vi "WebPublishing-DropIn.vi"(4 "Error In":errorcluster, 5 "Stop Occurrence":refnum<k4>, 6 "Mode (Snapshot)":enum16{"Snapshot", "Monitored", "Embedded"}(ring), 7 "VI Ref":refnum<vi>) -> (0 "Error Out":errorcluster, 1 "Web Server:Active":bool, 2 "URL":string, 3 "HTML File Name":path)   [LabVIEW 2016, in "CS++Utilities.lvlib"]
doc: "This VI will generate a Web Publishing HTML file for the Caller-VI in Web-Server file space to be viewed by remote Web-Browser.\n\nThis VI is used as drop-in. Simply connect an occurrence to stop this VI. It will clean up generated files.\n\n<b>Attention:</b> Library- and VI-Names should avoid any special charackters. They may be not recognizes by the Web-Publishing-Server."
uses:
  CS++Utilities.lvlib
panel:
  in  "Html_Code_Snapshot":string="<!DOCTYPE HTML PUBLIC \"-//W3C//DTD HTML 3.2 Draft//EN\">\n<HTML>\n<HEAD>\n<TITLE>WINDOW_TITLE</TITLE>\n</HEAD>\n<BODY >\n<H1>WINDOW_TITLE</H1>\n<IMG src=\"/.snap?SUBSTITUTE_VI_NAME\" alt=\"SUBSTITUTE_VI_NAME\" BORDER=1>\n<p>VI_DESCRIPTION</p>\n<p>HTML generated by CS++ WebPublishing-DropIn, H.Brand@gsi.de.</p>\n</BODY>\n</HTML>\n"
  in  "Html_Code_Monitor":string="<!DOCTYPE HTML PUBLIC \"-//W3C//DTD HTML 3.2 Draft//EN\">\n<HTML>\n<HEAD>\n<TITLE>WINDOW_TITLE</TITLE>\n<script language=\"javascript\">\n   <!-- \n   LVImages = new Array();\n   LVSrcs = new Array();\n   function LVSched(image, delay) {\n      LVImages[LVImages.length] = image;\n      LVSrcs[LVSrcs.length] = image.src;\n      setInterval(\"LVUpdate(\"+(LVImages.length-1)+\")\", delay);\n      image.onload='';\n   }\n   function LVUpdate(index) {\n      LVImages[index].src = LVSrcs[index] + '&' + Math.random();\n   }\n   //-->\n</script>\n</HEAD>\n<BODY >\n<H1>WINDOW_TITLE</H1>\n<IMG src=\"/.snap?SUBSTITUTE_VI_NAME\" alt=\"SUBSTITUTE_VI_NAME\" BORDER=1 onload=\"LVSched(this, 1000)\">\n<p>VI_DESCRIPTION</p>\n<p>HTML generated by CS++ WebPublishing-DropIn, H.Brand@gsi.de.</p>\n</BODY>\n</HTML>"
  in  "Html_Code_Embedded":string="<!DOCTYPE HTML PUBLIC \"-//W3C//DTD HTML 3.2 Draft//EN\">\n<HTML>\n<HEAD>\n<Script Language=\"JavaScript\">\nvar userAgent = navigator.userAgent;\nvar versionOffset = userAgent.indexOf(\"Chrome\");\n\nif (versionOffset != -1)\n{\n    var fullVersion = userAgent.substring(versionOffset+7);\n    var majorVersion = parseInt(''+fullVersion,10);\n    if (majorVersion >= 42)\n    {\n\tvar plugins = navigator.plugins;\n\tvar hasNIPlugin = false;\n\tfor (var i = 0; i < plugins.length; i++) {\n\t\tif (plugins[i].name.indexOf(\"National Instruments\") != -1) {\n\t\t\thasNIPlugin = true;\n\t\t}\n\t}\n\tif (hasNIPlugin == false) {\n        \tdocument.write('<strong><em>NI has detected that your ' +\n                               'browser might be blocking a plug-in.  '+\n                               'Visit ni.com/info and enter the following '+\n                               'Info Code for more information: '+\n                               'BlockedPlugin</em></strong>')\n\t}\n    }\n}\n</Script>\n<TITLE>WINDOW_TITLE</TITLE>\n</HEAD>\n<BODY >\n<H1>WINDOW_TITEL</H1>\n<p><TABLE BORDER=1 BORDERCOLOR = #000000><TR><TD>\n<OBJECT ID=\"LabVIEWControl\" CLASSID=\"CLSID:A40B0AD4-B50E-4E58-8A1D-8544233807B8\" WIDTH=PANEL_WIDTH HEIGHT=PANEL_HEIGHT CODEBASE=\"ftp://ftp.ni.com/support/labview/runtime/windows/2016/LVRTE2016min.exe\">\n<PARAM name=\"LVFPPVINAME\" value=\"SUBSTITUTE_VI_NAME\">\n<PARAM name=\"REQCTRL\" value=false>\n<EMBED SRC=\".LV_FrontPanelProtocol.rpvi160\" LVFPPVINAME=\"SUBSTITUTE_VI_NAME\" REQCTRL=false TYPE=\"application/x-labviewrpvi160\" WIDTH=PANEL_HEIGHT HEIGHT=PANEL_HEIGHT  PLUGINSPAGE=\"http://digital.ni.com/express.nsf/bycode/exck2m\">\n</EMBED>\n</OBJECT>\n</TD></TR></TABLE></p>\n<p>VI_DESCRIPTION</p>\n<p>HTML generated by CS++ WebPublishing-DropIn, H.Brand@gsi.de.</p>\n</BODY>\n</HTML>"
  in  "SHDocVw.IWebBrowser2":refnum<k7>
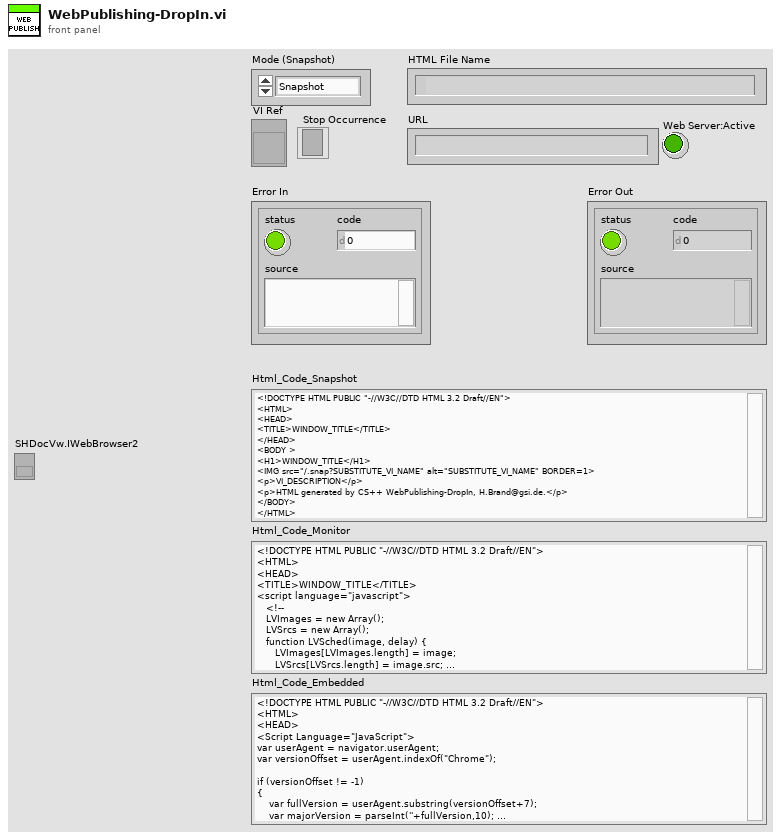
[diagram p1: front panel]
types:
  T1 = enum16{"open", "replace", "create", "open or create", "replace or create", "replace or create with confirmation"}
  T2 = typedef "LVRectTypeDef.ctl" = cluster{"Left":i16, "Top":i16, "Right":i16, "Bottom":i16}
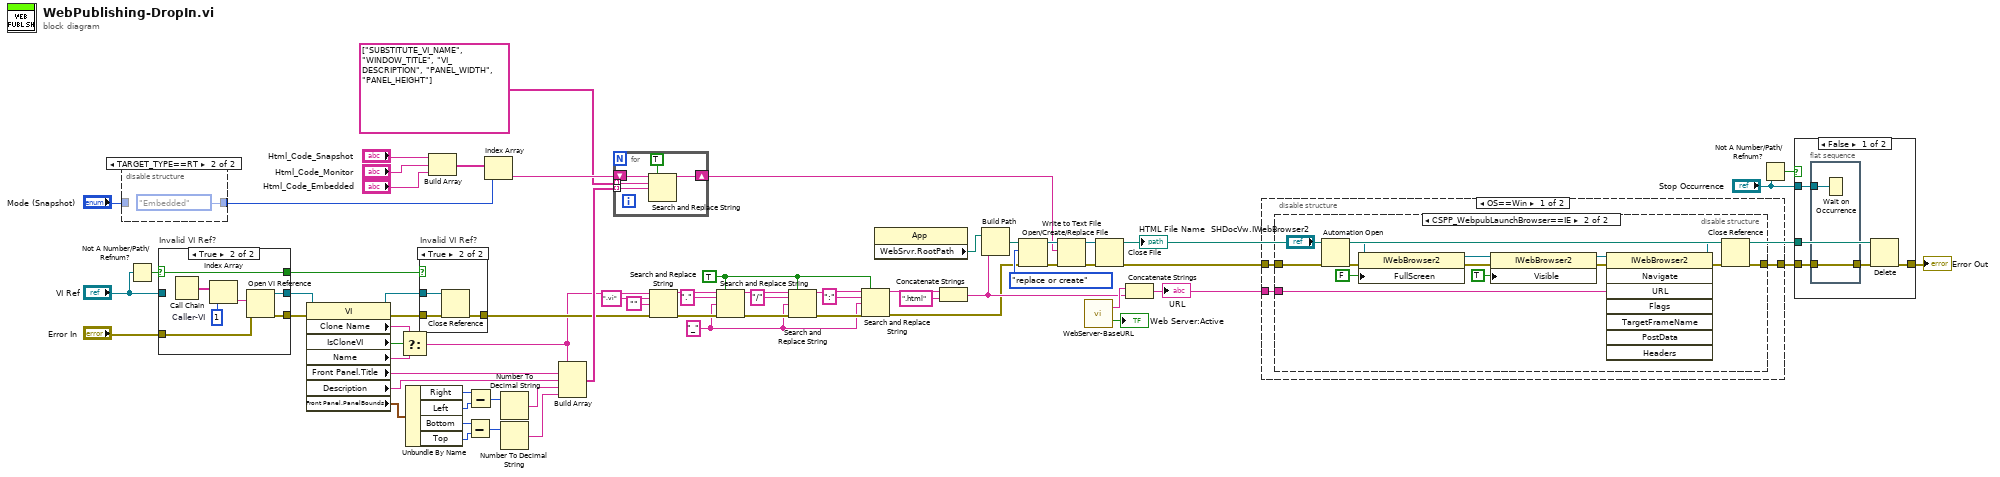
[diagram p0: block diagram]
diagram:
  w10 = TRUE ("replace all? (F)")
  w2 = "_"
  n1 = disable-structure shown="TARGET_TYPE==RT" {
    disable-tunnel: "Mode (Snapshot)" -> [w68 _]
    disable-tunnel: [w68 enum16{"Snapshot", "Monitored", "Embedded"}."Embedded" ("Mode (Snapshot)")] -> w26
    frame condition #0 (active) {
    }
    frame condition #1 {
    }
  }
  n2 = Not A Number/Path/Refnum?(number/path/refnum="VI Ref") -> (NaN/Path/Refnum?=w30:bool)
  n3 = case "Invalid VI Ref?" shown="True" w30 {
    selector: w30 -> [w70 w73]
    tunnel: [w72 w76] -> w67
    tunnel: [w71 w75] -> w61
    tunnel: "Error In" -> [w71 w74]
    tunnel: "VI Ref" -> [w72 _]
    tunnel: [w70 w73] -> w28
    frame False {
    }
    frame True {
      w79 = 1  # Caller-VI
      n4 = Call Chain() -> (call chain=w78:string[])
      n5 = Index Array(array=w78, index=w79) -> (element=w77:string)
      n6 = Open VI Reference(vi path=w77, error in (no error)=w74) -> (vi reference=w76:refnum<vi>, error out=w75:errorcluster)  [unwired: 4 in]
    }
  }
  n7 = property class="VI"(reference=w67, error in=w61) -> (reference out=w66:refnum<vi>, error out=w60:errorcluster, "Clone Name"=w45:string, "IsCloneVI"=w46:bool, "Name"=w44:string, "Front Panel.Title"=w23:string, "Description"=w22:string, "Front Panel.PanelBounds"=w20:T2)
  n8 = Select(t=w45, s=w46, f=w44) -> (s? t:f=w1:string)
  n9 = Unbundle By Name(w20) -> ("Right"=w19:i16, "Left"=w18:i16, "Bottom"=w17:i16, "Top"=w16:i16)
  n10 = case "Invalid VI Ref?" shown="True" w28 {
    tunnel: w66 -> [_ w83]
    tunnel: w60 -> [w80 w82]
    tunnel: [w80 w81] -> w5
    frame False {
    }
    frame True {
      n11 = Close Reference(reference=w83, error in (no error)=w82) -> (error out=w81:errorcluster)
    }
  }
  n12 = Build Array("Html_Code_Snapshot", "Html_Code_Monitor", "Html_Code_Embedded") -> (w52:string[])
  n13 = Subtract(x=w17, y=w16) -> (x-y=w13:i16)
  n14 = Subtract(x=w19, y=w18) -> (x-y=w15:i16)
  n15 = Index Array(array=w52, index=w26) -> (element=w51:string)
  n16 = Number To Decimal String(number=w13) -> (decimal integer string=w12:string)  [unwired: 1 in]
  n17 = Number To Decimal String(number=w15) -> (decimal integer string=w14:string)  [unwired: 1 in]
  n18 = Build Array(w1, w23, w22, w14, w12) -> (w24:string[])
  n19 = for {
    tunnel: string[] ["SUBSTITUTE_VI_NAME", "WINDOW_TITLE", "VI_DESCRIPTION", "PANEL_WIDTH", "PANEL_HEIGHT"] -> [w86] mode=indexing
    tunnel: w24 -> [w85] mode=indexing
    shift-right: [w84] -> w21
    shift-left: w51 -> [w87]
    n20 = Search and Replace String(replace all?=TRUE ("replace all? (F)"), input string=w87, search string=w86, replace string=w85) -> (result string=w84:string)  [unwired: 4 in, 3 out]
  }
  n21 = Search and Replace String(input string=w1, search string=".vi", replace string="", error in=w5) -> (result string=w3:string, error out=w4:errorcluster)  [unwired: 4 in, 2 out]
  n22 = Search and Replace String(replace all?=w10, input string=w3, search string=".", replace string=w2, error in=w4) -> (result string=w9:string, error out=w8:errorcluster)  [unwired: 3 in, 2 out]
  n23 = Search and Replace String(replace all?=w10, input string=w9, search string="/", replace string=w2, error in=w8) -> (result string=w32:string, error out=w31:errorcluster)  [unwired: 3 in, 2 out]
  n24 = Search and Replace String(replace all?=w10, input string=w32, search string=":", replace string=w2, error in=w31) -> (result string=w6:string, error out=w7:errorcluster)  [unwired: 3 in, 2 out]
  n25 = property class="App"() -> ("WebSrvr.RootPath"=w47:path)  [unwired: 2 in, 2 out]
  n26 = Concatenate Strings(w6, ".html") -> (w42:string)
  n27 = Build Path(base path=w47, name or relative path=w42) -> (appended path=w48:path)
  n28 = Open/Create/Replace File(file path (use dialog)=w48, error in=w7, operation (0:open)=T1."replace or create") -> (refnum out=w65:refnum<file>, error out=w63:errorcluster)  [unwired: 3 in, 1 out]
  n29 = Write to Text File(file (use dialog)=w65, text=w21, error in=w63) -> (refnum out=w64:refnum<file>, error out=w62:errorcluster)  [unwired: 1 in, 1 out]
  n30 = call "WebServer-BaseURL.vi"() -> ("Web Server:Active"=→"Web Server:Active":bool, "Web-Server:Base-URL"=w43:string)
  n31 = Close File(refnum=w64, error in=w62) -> (path=w38:path, error out=w56:errorcluster)
  "HTML File Name" <- w38
  n32 = Concatenate Strings(w43, w42) -> (w41:string)
  "URL" <- w41
  n33 = disable-structure shown="OS==Win" {
    disable-tunnel: w56 -> [w91 w106]
    disable-tunnel: w41 -> [w90 _]
    disable-tunnel: [w89 w106] -> w39
    frame condition #0 (active) {
      n34 = disable-structure shown="CSPP_WebpubLaunchBrowser==IE" {
        disable-tunnel: w91 -> [_ w105]
        disable-tunnel: w90 -> [_ w104]
        disable-tunnel: [_ w103] -> w89
        frame condition #0 {
        }
        frame condition #1 (active) {
          n35 = Automation Open(error in (no error)=w105, Automation Refnum="SHDocVw.IWebBrowser2") -> (Automation Refnum=w96:refnum<k7>, error out=w97:errorcluster)  [unwired: 2 in]
          n36 = property class="IWebBrowser2"(reference=w96, error in=w97, "FullScreen"=FALSE) -> (reference out=w101:refnum<k7>, error out=w102:errorcluster)
          n37 = property class="IWebBrowser2"(reference=w101, error in=w102, "Visible"=TRUE) -> (reference out=w94:refnum<k7>, error out=w95:errorcluster)
          n38 = invoke class="IWebBrowser2" method="Navigate"(reference=w94, error in=w95, "URL"=w104) -> (reference out=w92:refnum<k7>, error out=w93:errorcluster)  [unwired: 5 in, 6 out]
          n39 = Close Reference(reference=w92, error in (no error)=w93) -> (error out=w103:errorcluster)
        }
      }
    }
    frame condition #1 {
    }
  }
  n40 = Not A Number/Path/Refnum?(number/path/refnum="Stop Occurrence") -> (NaN/Path/Refnum?=w35:bool)
  n41 = case shown="False" w35 {
    tunnel: w39 -> [w110 w114]
    tunnel: w38 -> [w109 _]
    tunnel: [w108 w114] -> w37
    tunnel: "Stop Occurrence" -> [w107 _]
    frame False {
      n42 = flat-sequence {
        tunnel: [w113] -> w111
        tunnel: w110 -> [w113]
        tunnel: w107 -> [w112]
        frame #0 {
          n43 = Wait on Occurrence(2:w112) -> ()  [unwired: 2 in, 1 out]
        }
      }
      n44 = Delete(path (use dialog)=w109, error in=w111) -> (error out=w108:errorcluster)  [unwired: 3 in, 2 out]
    }
    frame True {
    }
  }
  "Error Out" <- w37
